vi "CRD HF v3.vi"   [LabVIEW 2015]
uses:
  <vilib>/rvi/eio/common/nirviEmuClasses.ctl
  <vilib>/rvi/Emulation/niFpgaGetClockAttributes.vi
  <vilib>/rvi/Emulation/niFpgaSctlEmulationGetInTimedLoop.vi
  <vilib>/rvi/Emulation/niFpgaEmulationReportErrorSimple.vi
  <vilib>/rvi/Emulation/niFpgaEmulationIsFPGAContextNoSignature.vi
  <vilib>/rvi/DataTransferAndStorage/Container/Common/niFpgaContainerGetUniqueNameForEmu.vi
  <vilib>/rvi/Memory/Memory_Emulation/niFpgaMemoryEmulationCacheClearOnFirstRun.vi
  <vilib>/rvi/Memory/Memory_Emulation/nirvimemoryEmulationManagerCache_MakeExclusive.vi
  <vilib>/rvi/Memory/Memory_Emulation/niFpgaMemoryEmulationValidateCache.vi
  <vilib>/rvi/Memory/Memory_Emulation/nirvimemoryEmulationManagerCache_InsertValue.vi
  <vilib>/Utility/error.llb/Clear Errors.vi
  <vilib>/rvi/Memory/Memory_Emulation/nirvimemoryEmulationManagerCache_ReleaseExclusive.vi
  <vilib>/rvi/Memory/Memory_Emulation/nirvimemoryEmulationManagerCache_GetValue.vi
  <vilib>/rvi/Memory/Memory_Emulation/nirvimemoryEmulationManagerCache_SetValue.vi
  <vilib>/rvi/Emulation/niFpgaProcessEmulError.vi
  <vilib>/rvi/Emulation/niFpgaCriticalErrorInLSC.vi
  <vilib>/rvi/eio/common/nirviEmuTemplateMethod_errors.vi
  <vilib>/rvi/errors/niFpgaSetErrorForExecOnDevCompSimple.vi
  <vilib>/rvi/eio/common/nirviEmuReportErrorAndStop.vi
  <vilib>/rvi/FIFO/Fifo_Resource/nirvififoEmulationSetSize.vi
  <vilib>/rvi/FIFO/Fifo_Resource/nirviFifoEmulationQueueMgr.vi
  <instcachedir>/0/nirviFifoEmulationQueueMgr_E5CAEC123FF24DC58D834DCA3CDAA9B5.lvgen/nirviFifoEmulationQueueMgr_E5CAEC123FF24DC58D834DCA3CDAA9B5_001.vi
  <vilib>/rvi/FIFO/Fifo_Resource/nirvififoEmulationCreateLock.vi
  <vilib>/rvi/FIFO/Fifo_Resource/nirvififoEmulationObtainLock.vi
  <vilib>/rvi/FIFO/Fifo_Resource/nirvififoEmulationReleaseLock.vi
  <vilib>/rvi/occurrence/nirviWaitOnOccurrenceBase.vi
  <vilib>/rvi/errors/nirviReportUnexpectedCaseInternalError.vi
  <vilib>/rvi/errors/nirviReportUnexpectedCaseInternalError (U32).vi
  <vilib>/rvi/FIFO/Fifo_Resource/nirvififoEmulationDetermineInputValidOut.vi
  <vilib>/rvi/DataTransferAndStorage/Container/XNode/niFpgaContainer.xnode
  <vilib>/rvi/DataTransferAndStorage/Register/Emulation/niFpgaRegisterEmulation.vi
  <vilib>/eio/EIOGrowableMethodNode/genericMethod/EIOGrowableMethodNode.xnode
  <vilib>/rvi/eio/nirviEIOMethodImplementation/nirviEIOMethodImplementation.xnode
  <vilib>/rvi/eio/nirviErrorMerge/nirviErrorMerge.xnode
  <vilib>/eio/EIONode/EIONode.xnode
  <vilib>/rvi/FIFO/Fifo_Resource/nirvififoEmulationRead.vi
  <vilib>/rvi/FIFO/Fifo_Resource/nirvififoEmulationWrite.vi
types:
  T1 = typedef "nirviEmuClasses.ctl" = enum16{"IO Read", "IO Write", "Method", "Property Read", "Property Write"}
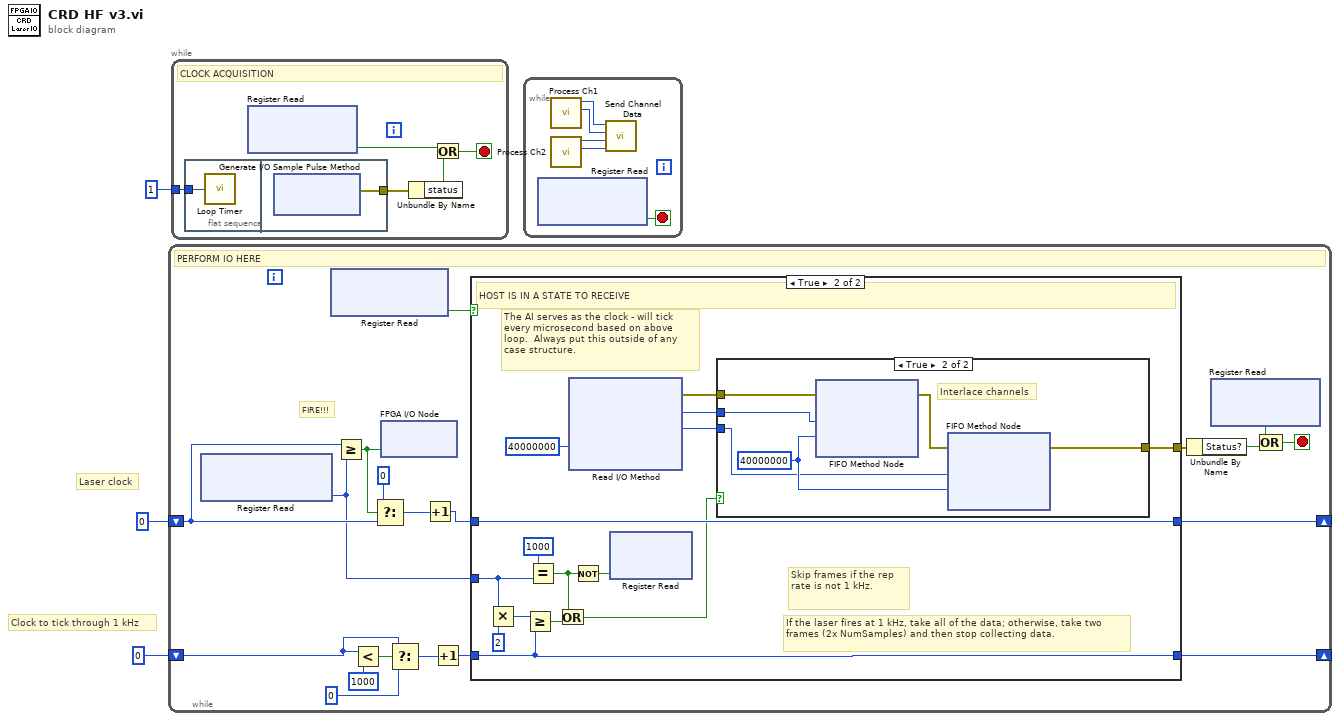
[diagram p0: block diagram]
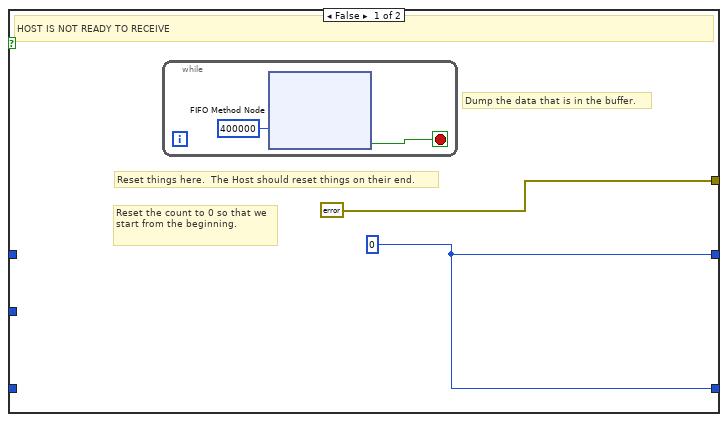
[diagram p2: hidden frame]
diagram:
  # "Laser clock"
  # "Clock to tick through 1 kHz"
  n1 = while {
    shift-right: [w16] -> _
    shift-left: u16 0 ("Number of Samples") -> [w17]
    shift-right: [w7] -> _
    shift-left: u16 0 ("Number of Samples") -> [w4]
    stop <- w6 stop-if-true
    # "FIRE!!!"
    # "PERFORM IO HERE"
    n2 = xnode ("Register Read")() -> ("Data"=w10:u16)  [unwired: 1 in, 1 out]
    n3 = xnode ("Register Read")() -> ("Data"=w13:bool)  [unwired: 1 in, 1 out]
    n4 = Greater Or Equal?(x=w17, y=w10) -> (x >= y?=w19:bool)
    n5 = Less?(x=w4, y=u16 1000) -> (x < y?=w9:bool)
    n6 = Select(t=u16 0 ("Number of Samples"), s=w19, f=w17) -> (s? t:f=w15:u16)
    n7 = xnode "FPGA I/O Node"("CRDS"=w19) -> ()  [unwired: 1 in, 1 out]
    n8 = Select(t=w4, s=w9, f=u16 0 ("Number of Samples")) -> (s? t:f=w12:u16)
    n9 = Increment(x=w15) -> (x+1=w14:u16)
    n10 = Increment(x=w12) -> (x+1=w8:u16)
    n11 = case shown="True" w13 {
      tunnel: [errorcluster {"Status?"=FALSE, "Code"=0, "Source"=""} ("error out") w27] -> w20
      tunnel: w14 -> [_ w41]
      tunnel: [w23 w41] -> w16
      tunnel: w10 -> [_ w37]
      tunnel: w8 -> [_ w32]
      tunnel: [w23 w32] -> w7
      frame False {
        w23 = u16 0 ("Number of Samples")
        # "Dump the data that is in the buffer."
        # "Reset things here.  The Host should reset things on their end."
        # "Reset the count to 0 so that we start from the beginning."
        # "HOST IS NOT READY TO RECEIVE"
        n12 = while {
          stop <- w26 stop-if-true
          n13 = xnode ("FIFO Method Node")("Timeout"=400000) -> ("Timed Out?"=w26:bool)  [unwired: 1 in, 2 out]
        }
      }
      frame True {
        # "The AI serves as the clock - will tick every microsecond based on above loop.  Always put this outside of any case structure."
        # "Skip frames if the rep rate is not 1 kHz."
        # "If the laser fires at 1 kHz, take all of the data; otherwise, take two frames (2x NumSamples) and then stop collecting data."
        # "HOST IS IN A STATE TO RECEIVE"
        n14 = Multiply(x=w37, y=u16 2) -> (x*y=w35:u16)
        n15 = Greater Or Equal?(x=w35, y=w32) -> (x >= y?=w34:bool)
        n16 = Equal?(x=u16 1000, y=w37) -> (x = y?=w39:bool)
        n17 = Or(x=w39, y=w34) -> (x .or. y?=w33:bool)
        n18 = xnode "Read I/O Method"("Timeout"=40000000) -> ("error out"=w29:errorcluster, "CRD Las Ch 1"=w30:i16, "CRD Las Ch 2"=w28:i16)  [unwired: 3 in, 3 out]
        n19 = Not(x=w39) -> (.not. x?=w38:bool)
        n20 = xnode ("Register Read")("Data"=w38) -> ()  [unwired: 1 in, 1 out]
        n21 = case shown="True" w33 {
          tunnel: w30 -> [_ w156]
          tunnel: w29 -> [w150 w155]
          tunnel: w28 -> [_ w153]
          tunnel: [w150 w151] -> w27
          frame False {
          }
          frame True {
            w154 = 40000000 ("Timeout")
            # "Interlace channels"
            n22 = xnode ("FIFO Method Node")("Element"=w156, "Timeout"=w154, "error in (no error)"=w155) -> ("error out"=w152:errorcluster)  [unwired: 1 in, 2 out]
            n23 = xnode ("FIFO Method Node")("Element"=w153, "Timeout"=w154, "error in (no error)"=w152) -> ("error out"=w151:errorcluster)  [unwired: 1 in, 2 out]
          }
        }
      }
    }
    n24 = Unbundle By Name(w20) -> ("Status?"=w22:bool)
    n25 = xnode ("Register Read")() -> ("Data"=w18:bool)  [unwired: 1 in, 1 out]
    n26 = Compound Arithmetic op=OR(w18, w22) -> (w6:bool)
  }
  n27 = while {
    tunnel: u32 1 ("Sample Period (uSec)") -> [w161]
    stop <- w157 stop-if-true
    # "CLOCK ACQUISITION"
    n28 = flat-sequence {
      tunnel: w161 -> [w162]
      tunnel: [w163] -> w160
      frame #0 {
        n29 = call "Loop Timer"("Count(uSec)"=w162) -> ()  [unwired: 1 out]
      }
      frame #1 {
        n30 = xnode "Generate I/O Sample Pulse Method"() -> ("error out"=w163:errorcluster)  [unwired: 2 in, 1 out]
      }
    }
    n31 = xnode ("Register Read")() -> ("Data"=w159:bool)  [unwired: 1 in, 1 out]
    n32 = Unbundle By Name(w160) -> ("status"=w158:bool)
    n33 = Or(x=w159, y=w158) -> (x .or. y?=w157:bool)
  }
  n34 = while {
    stop <- w212 stop-if-true
    n35 = xnode ("Register Read")() -> ("Data"=w212:bool)  [unwired: 1 in, 1 out]
    n36 = call "Process Ch1.vi"() -> ("Max1"=w210:u32, "Max0"=w211:u32)  [unwired: 10 in]
    n37 = call "Process Ch2.vi"() -> ("Max4"=w208:u32, "Max3"=w209:u32)  [unwired: 10 in]
    n38 = call "Send Channel Data.vi"("Max3"=w208, "Max2"=w209, "Max1"=w210, "Max0"=w211) -> ()  [unwired: 8 in]
  }
